vi "GetMainQueue.vi"(8 "error in (no error)":errorcluster) -> (0 "error out":errorcluster, 3 "queue out":refnum<queue>)   [LabVIEW 2013]
uses:
  QueueInstruction.ctl
  QueueSubsystem.ctl
  QueueAction.ctl
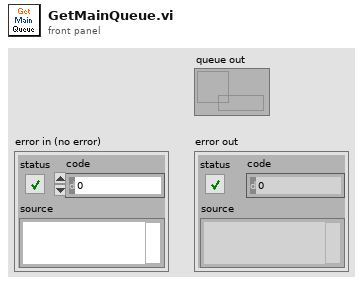
[diagram p1: front panel]
types:
  T1 = typedef "QueueInstruction.ctl" = cluster{"Data":variant, "Subsystem":T2, "Action":T3}
  T2 = typedef "QueueSubsystem.ctl" = enum16{"Drive", "SonicShifter", "Kicker", "FirePneumatic", "Roller", "Clapper", "RollerRelay"}
  T3 = typedef "QueueAction.ctl" = enum16{"Init", "SetValue", "Disable"}
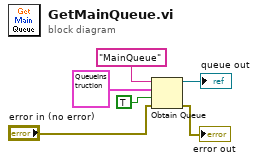
[diagram p0: block diagram]
diagram:
  n1 = Obtain Queue(name (unnamed)="MainQueue", element data type=T1 {"Data"=variant, "Subsystem"=enum."SonicShifter", "Action"=enum."Init"}, create if not found? (T)=TRUE, error in (no error)="error in (no error)") -> (queue out=→"queue out":refnum<queue>, error out=→"error out":errorcluster)  [unwired: 1 in, 1 out]
